vi "SubVI ReactionWheel.vi"(10 "Roll angle":dbl, 11 "Roll reference":dbl) -> (2 "Output PWM":dbl)   [LabVIEW 2021]
uses:
  <vilib>/myRIO/Instrument Drivers/Onboard IO/DIO/typedefs/DIO Reference.ctl
  <vilib>/myRIO/Common/Instrument Driver Framework/Utilities/typedefs/myRIO Generic Hardware Reference.ctl
  <vilib>/myRIO/Common/Instrument Driver Framework/Utilities/typedefs/Hardware Version Enum.ctl
  <vilib>/myRIO/Common/Instrument Driver Framework/Utilities/typedefs/myRIO v1.0 Reference.ctl
  <vilib>/myRIO/Common/Instrument Driver Framework/Utilities/typedefs/Generic FPGA Reference.ctl
  <vilib>/myRIO/Common/Instrument Driver Framework/myRIO v1.0/DIO/typedefs/DIO Channels List.ctl
  <vilib>/myRIO/Common/Instrument Driver Framework/myRIO v1.0/DIO/typedefs/DIO Channels Enum.ctl
  <vilib>/userdefined/High Color/nirio_resource_hc.ctl
  <vilib>/myRIO/Instrument Drivers/Onboard IO/PWM/typedefs/PWM Reference.ctl
  <vilib>/myRIO/Common/Instrument Driver Framework/myRIO v1.0/PWM/typedefs/PWM Channels Enum.ctl
  <vilib>/myRIO/Instrument Drivers/Onboard IO/PWM/typedefs/PWM Configuration.ctl
  <vilib>/myRIO/Common/Instrument Driver Framework/Utilities/vis/Is FPGA Ref Available.vi
  <vilib>/myRIO/Common/Instrument Driver Framework/myRIO v1.0/DIO/vis/myRIO v1.1 Open DIO.vi
  <vilib>/myRIO/Instrument Drivers/Onboard IO/DIO/vis/Write.vi
  <vilib>/myRIO/Common/Instrument Driver Framework/myRIO v1.0/PWM/vis/myRIO v1.1 Open PWM.vi
  <vilib>/myRIO/Instrument Drivers/Onboard IO/PWM/vis/Set Duty Cycle and Frequency.vi
  <vilib>/myRIO/Common/Instrument Driver Framework/Utilities/vis/Validate Channels.vi
  <vilib>/myRIO/Common/Instrument Driver Framework/myRIO v1.0/DIO/vis/myRIO v1.0 Reserve DIO.vi
  <vilib>/myRIO/Common/Instrument Driver Framework/myRIO v1.0/PWM/vis/myRIO v1.0 Reserve PWM.vi
  <vilib>/myRIO/Common/Instrument Driver Framework/myRIO v1.0/Resource Manager/vis/myRIO v1.0 Reserve Channel List.vi
  <vilib>/myRIO/Common/Instrument Driver Framework/myRIO v1.0/DIO/vis/myRIO v1.0 Build MUX Configuration DIO.vi
  <vilib>/myRIO/Common/Instrument Driver Framework/myRIO v1.0/PWM/vis/myRIO v1.0 Build MUX Configuration PWM.vi
  <vilib>/myRIO/Common/Instrument Driver Framework/myRIO v1.0/Resource Manager/vis/myRIO v1.0 Reserve Channel.vi
  <vilib>/myRIO/Common/Instrument Driver Framework/myRIO v1.0/Resource Manager/vis/myRIO v1.0 Unreserve Channel.vi
  <vilib>/myRIO/Common/Instrument Driver Framework/myRIO v1.0/Resource Manager/vis/myRIO v1.0 Create Configuration List.vi
  <vilib>/myRIO/Common/Instrument Driver Framework/myRIO v1.0/Resource Manager/vis/myRIO v1.0 Build Mutex Name.vi
  <vilib>/addons/control/pid/pid.llb/PID (DBL).vi
  <vilib>/Utility/VariantDataType/GetNumericInfo.vi
  <vilib>/Utility/error.llb/Error Cluster From Error Code.vi
  <vilib>/myRIO/Common/Instrument Driver Framework/myRIO v1.0/myRIO v1.1 Open.vi
  <vilib>/myRIO/Common/Instrument Driver Framework/Utilities/vis/IO Manager.vi
  <vilib>/myRIO/Common/Instrument Driver Framework/Utilities/vis/Configuration Manager.vi
  <vilib>/myRIO/Common/Instrument Driver Framework/myRIO v1.0/Resource Manager/vis/myRIO v1.0 Configure IO.vi
  <vilib>/myRIO/Common/Instrument Driver Framework/myRIO v1.0/myRIO v1.0 Close.vi
  <vilib>/myRIO/Common/Instrument Driver Framework/myRIO v1.0/DIO/vis/myRIO v1.0 Write DIO.vi
  <vilib>/myRIO/Common/Instrument Driver Framework/myRIO v1.0/PWM/vis/myRIO v1.0 Write PWM.vi
  <vilib>/myRIO/Express VI/Onboard Devices/LED/LED Express VI.xnode
  <vilib>/myRIO/Instrument Drivers/Onboard IO/DIO/vis/myRIO DIO Open.xnode
  <vilib>/myRIO/Express VI/Onboard IO/PWM/PWM Express VI.xnode
  <vilib>/myRIO/Instrument Drivers/Onboard IO/PWM/vis/myRIO PWM Open.xnode
  <vilib>/myRIO/Instrument Drivers/Onboard IO/PWM/PWM.lvlib
  <vilib>/addons/control/pid/NI_PID_pid.lvlib
  <vilib>/myRIO/Instrument Drivers/Onboard IO/DIO/DIO.lvlib
panel:
  in  "LED indicators off/on":bool
  in  "Outer deadzone off/on":bool
  in  "Inner deadzone off/on":bool
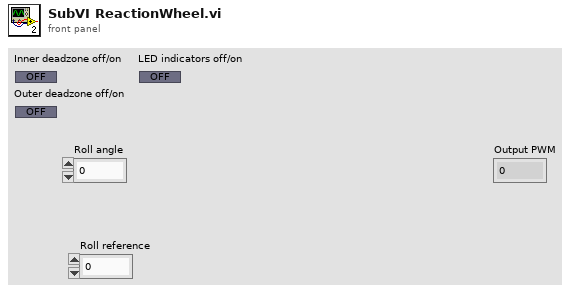
[diagram p1: front panel]
types:
  T1 = typedef "DIO.lvlib/DIO Reference.ctl" = cluster{"myRIO Reference":T2, "DIO Channels List":T6}
  T2 = typedef "myRIO Generic Hardware Reference.ctl" = cluster{"myRIO Model":T3, "myRIO Hardware Reference":T4}
  T3 = typedef "Hardware Version Enum.ctl" = enum16{"Unknown", "myRIO-1900", "myRIO-1950", "roboRIO", "NI ELVIS RIO CM", "ELVIS III"}
  T4 = typedef "myRIO v1.0 Reference.ctl" = cluster{"Generic FPGA Reference":T5, "Allow multiple opens":bool}
  T5 = typedef "Generic FPGA Reference.ctl" = refnum<k20>
  T6 = typedef "DIO Channels List.ctl" = T7[]
  T7 = typedef "DIO Channels Enum.ctl" = enum16{"Not Connected", "C/DIO0", "C/DIO1", "C/DIO2", "C/DIO3", "C/DIO4", "C/DIO5", "C/DIO6", "C/DIO7", "A/DIO0", "A/DIO1", "A/DIO2", "A/DIO3", "A/DIO4", "A/DIO5", "A/DIO6", "A/DIO7", "A/DIO8", "A/DIO9", "A/DIO10", "A/DIO11", "A/DIO12", "A/DIO13", "A/DIO14", "A/DIO15", "A/DIO16", "A/DIO17", "A/DIO18", "A/DIO19", "B/DIO0", "B/DIO1", "B/DIO2", "B/DIO3", "B/DIO4", "B/DIO5", "B/DIO6", "B/DIO7", "B/DIO8", "B/DIO9", "B/DIO10", "B/DIO11", "B/DIO12", "B/DIO13", "B/DIO14", "B/DIO15", "B/DIO16", "B/DIO17", "B/DIO18", "B/DIO19", "LED0", "LED1", "LED2", "LED3", "Button0", "DIO/DIO0", "DIO/DIO1", "DIO/DIO2", "DIO/DIO3", "DIO/DIO4", "DIO/DIO5", "DIO/DIO6", "DIO/DIO7", "DIO/DIO8", "DIO/DIO9", "SPI/CS0", "SPI/CS1", "SPI/CS2", "SPI/CS3", "LED RADIO (Green)", "LED RADIO (Red)", "LED COMM (Green)", "LED COMM (Red)", "LED MODE (Green)", "LED MODE (Red)"}
  T8 = typedef "nirio_resource_hc.ctl" = tag
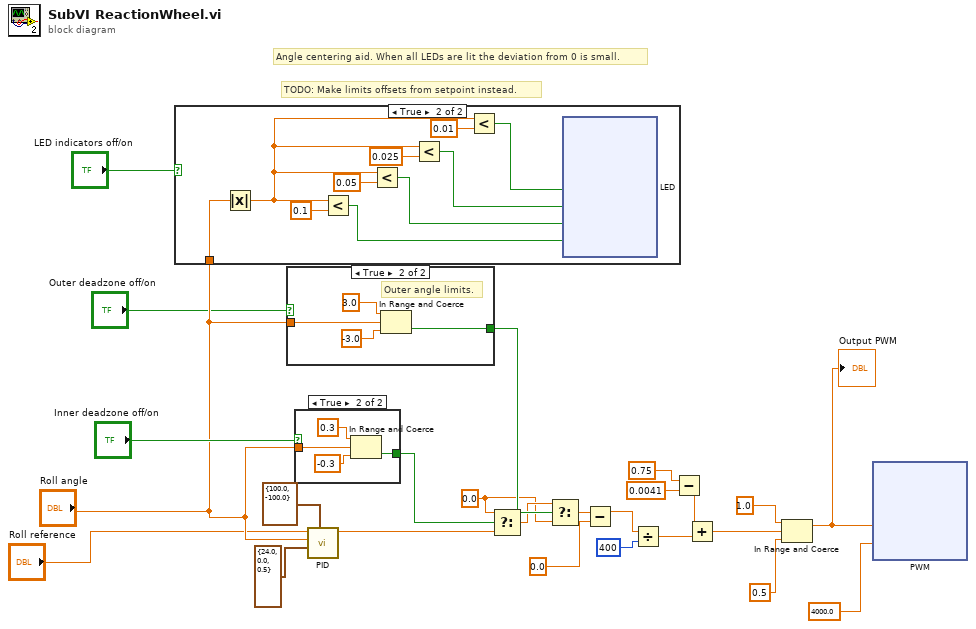
[diagram p0: block diagram]
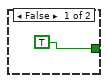
[diagram p3: hidden frame]
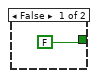
[diagram p4: hidden frame]
diagram:
  w10 = 0.0
  # "TODO: Make limits offsets from setpoint instead."
  # "Angle centering aid. When all LEDs are lit the deviation from 0 is small."
  n1 = case shown="True" "LED indicators off/on" {
    tunnel: "Roll angle" -> [_ w26]
    frame False {
    }
    frame True {
      n2 = Absolute Value(x=w26) -> (abs(x)=w27:dbl)
      n3 = Less?(x=w27, y=0.1) -> (x < y?=w35:bool)
      n4 = Less?(x=w27, y=0.05) -> (x < y?=w32:bool)
      n5 = Less?(x=w27, y=0.025) -> (x < y?=w30:bool)
      n6 = Less?(x=w27, y=0.01) -> (x < y?=w28:bool)
      n7 = xnode "LED"("LED0"=w28, "LED1"=w30, "LED2"=w32, "LED3"=w35) -> ()  [unwired: 1 in, 1 out]
    }
  }
  n8 = case shown="True" "Outer deadzone off/on" {
    tunnel: [TRUE w76] -> w13
    tunnel: "Roll angle" -> [_ w75]
    frame False {
    }
    frame True {
      # "Outer angle limits."
      n9 = In Range and Coerce(upper limit=3.0 ("Angle deadzone upper limit"), x=w75, lower limit=-3.0 ("Angle deadzone lower limit")) -> (In Range?=w76:bool)  [unwired: 1 out]
    }
  }
  n10 = case shown="True" "Inner deadzone off/on" {
    tunnel: [FALSE w83] -> w15
    tunnel: "Roll angle" -> [_ w82]
    frame False {
    }
    frame True {
      n11 = In Range and Coerce(upper limit=0.3 ("Angle deadzone upper limit"), x=w82, lower limit=-0.3 ("Angle deadzone lower limit")) -> (In Range?=w83:bool)  [unwired: 1 out]
    }
  }
  n12 = call-poly <vilib>:"PID.vi"("output range"=cluster{"Maximum":dbl, "Minimum":dbl} {"Maximum"=100.0, "Minimum"=-100.0} ("PID output range"), "PID gains"=cluster{"P":dbl, "I":dbl, "D":dbl} {"P"=24.0, "I"=0.0, "D"=0.5}, "process variable"="Roll angle", "setpoint"="Roll reference") -> ("output"=w16:dbl)  [unwired: 6 in, 1 out]
  n13 = Select(t=w10, s=w15, f=w16) -> (s? t:f=w11:dbl)
  n14 = Select(t=w11, s=w13, f=w10) -> (s? t:f=w12:dbl)
  n15 = Subtract(x=w12, y=0.0) -> (x-y=w9:dbl)
  n16 = Divide(x=w9, y=400) -> (x/y=w19:dbl)
  n17 = Subtract(x=0.75, y=0.0041) -> (x-y=w7:dbl)
  n18 = Add(x=w7, y=w19) -> (x+y=w24:dbl)
  n19 = In Range and Coerce(upper limit=1.0 ("Max PWM"), x=w24, lower limit=0.5 ("Min PWM")) -> (coerced(x)=w3:dbl)  [unwired: 1 out]
  "Output PWM" <- w3
  n20 = xnode "PWM"("Duty Cycle"=w3, "Frequency [Hz]"=4000.0 ("PWMfrekvens")) -> ()  [unwired: 1 in, 1 out]
